vi "Create.vi"(8 "error in (no error)":errorcluster, 10 "thread configuration":T1={"core"={"processor"=-2, "priority offset"=0}, "component settings"=[], "transfer groups"=[]}, 11 "Thread Configuration in":refnum<class "Thread Configuration.lvclass">) -> (0 "error out":errorcluster, 3 "Thread Configuration out":refnum<class "Thread Configuration.lvclass">)   [LabVIEW 2019, in "DSF Core.lvlib" / "Thread Configuration.lvclass"]
uses:
  Thread Configuration.lvclass
  C:/Dev/GitHub/niveristand-data-sharing-framework-custom-device/Core/Classes/Configuration/Core/Core Configuration.lvclass
  Typedefs/DSF Engine Plugin Thread Configuration.ctl
  Typedefs/Core Thread Configuration.ctl
  Typedefs/DSF Settings Info.ctl
  Typedefs/DSF Engine Transfer Group Configuration.ctl
  Typedefs/Core Group Configuration.ctl
  Typedefs/DSF Direction.ctl
  Typedefs/DSF Timing Info.ctl
  Typedefs/DSF Timeout Behavior.ctl
  Typedefs/DSF Engine Transfer Configuration.ctl
  Typedefs/Core Transfer Configuration.ctl
  Typedefs/DSF Engine Channel Configuration.ctl
  Typedefs/Core Channel Configuration.ctl
  Typedefs/DSF Data Type.ctl
  Thread Configuration.lvclass/Thread Configuration.ctl
  Group/Group Configuration.lvclass
  Core Configuration.lvclass
  DSF Core.lvlib
  Channel/Channel Configuration.lvclass
  Transfer/Transfer Configuration.lvclass
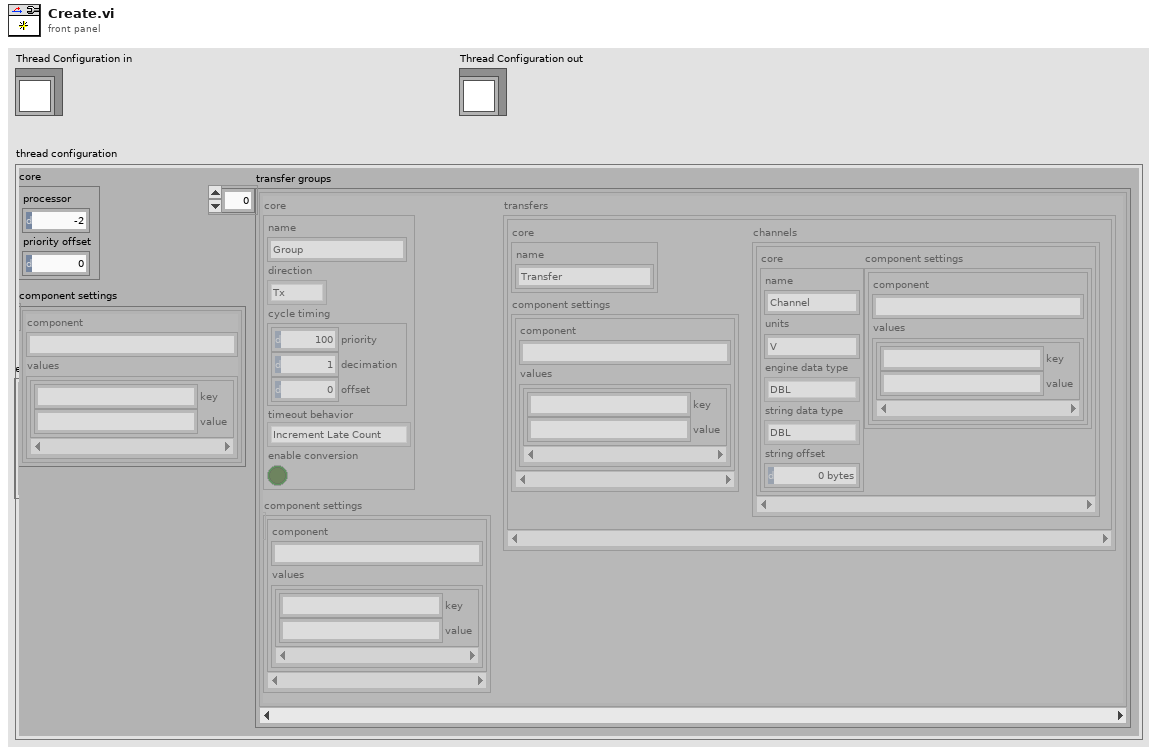
[diagram p1: front panel]
types:
  T1 = typedef "DSF Core.lvlib/DSF Engine Plugin Thread Configuration.ctl" = cluster{"core":T2, "component settings":T3[], "transfer groups":T4[]}
  T2 = typedef "DSF Core.lvlib/Thread Configuration.lvclass/Core Thread Configuration.ctl" = cluster{"processor":i32, "priority offset":i16}
  T3 = typedef "DSF Core.lvlib/DSF Settings Info.ctl" = cluster{"component":string, "values":cluster{"key":string, "value":string}[]}
  T4 = typedef "DSF Core.lvlib/DSF Engine Transfer Group Configuration.ctl" = cluster{"core":T5, "component settings":T3[], "transfers":T9[]}
  T5 = typedef "DSF Core.lvlib/Group Configuration.lvclass/Core Group Configuration.ctl" = cluster{"name":string, "direction":T6, "cycle timing":T7, "timeout behavior":T8, "enable conversion":bool}
  T6 = typedef "DSF Core.lvlib/DSF Direction.ctl" = enum8{"Tx", "Rx"}
  T7 = typedef "DSF Core.lvlib/DSF Timing Info.ctl" = cluster{"priority":u64, "decimation":u64, "offset":u64}
  T8 = typedef "DSF Core.lvlib/DSF Timeout Behavior.ctl" = enum8{"Increment Late Count", "Throw Error"}
  T9 = typedef "DSF Core.lvlib/DSF Engine Transfer Configuration.ctl" = cluster{"core":T10, "component settings":T3[], "channels":T11[]}
  T10 = typedef "DSF Core.lvlib/Transfer Configuration.lvclass/Core Transfer Configuration.ctl" = cluster{"name":string}
  T11 = typedef "DSF Core.lvlib/DSF Engine Channel Configuration.ctl" = cluster{"core":T12, "component settings":T3[]}
  T12 = typedef "DSF Core.lvlib/Channel Configuration.lvclass/Core Channel Configuration.ctl" = cluster{"name":string, "units":string, "engine data type":T13, "string data type":T13, "string offset":u64}
  T13 = typedef "DSF Core.lvlib/DSF Data Type.ctl" = enum8{"Bool", "SGL", "DBL", "I8", "I16", "I32", "I64", "U8", "U16", "U32", "U64"}
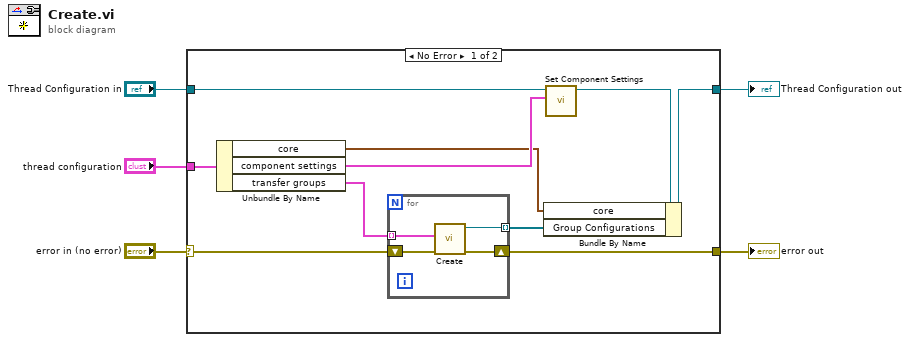
[diagram p0: block diagram]
diagram:
  n1 = case shown="No Error" "error in (no error)" {
    selector: "error in (no error)" -> [w14 w21]
    tunnel: [w11 w21] -> w4
    tunnel: [w15 w20] -> w2
    tunnel: "Thread Configuration in" -> [w7 w20]
    tunnel: "thread configuration" -> [w8 _]
    frame No Error {
      n2 = Unbundle By Name(w8) -> ("core"=w6:T2, "component settings"=w9:T3[], "transfer groups"=w13:T4[])
      n3 = for {
        shift-right: [w17] -> w11
        shift-left: w14 -> [w19]
        tunnel: w13 -> [w18] mode=indexing
        tunnel: [w16] -> w12 mode=indexing
        n4 = call "Create.vi"("error in (no error)"=w19, "group configuration"=w18) -> ("error out"=w17:errorcluster, "Group Configuration out"=w16:refnum<class "Group Configuration.lvclass">)  [unwired: 8 in]
      }
      n5 = call "Set Component Settings.vi"("component settings"=w9, "Runtime Configuration in"=w7) -> ("Runtime Configuration out"=w10:refnum<class "Thread Configuration.lvclass">)  [unwired: 8 in, 1 out]
      n6 = Bundle By Name(cluster=w10, "core"=w6, "Group Configurations"=w12) -> (w15:refnum<class "Thread Configuration.lvclass">)
    }
    frame Error {
    }
  }
  "error out" <- w4
  "Thread Configuration out" <- w2
